vi "Update Armed.vi"(8 "error in (no error)":errorcluster, 10 "Armed":bool, 11 "Monitor-Pulse in":refnum<class "LabActor.lvclass">) -> (0 "error out":errorcluster, 3 "Monitor-Pulse out":refnum<class "LabActor.lvclass">)   [LabVIEW 2016, in "LabActor.lvclass"]
uses:
  LabActor.lvclass
  C:/github/LabActor/Controllers/Application Controller/Application Controller.lvclass
  Controllers/Application Controller/Application Controller.lvclass/Application Controller.ctl
  Controllers/Application Controller/Read Armed ref.vi
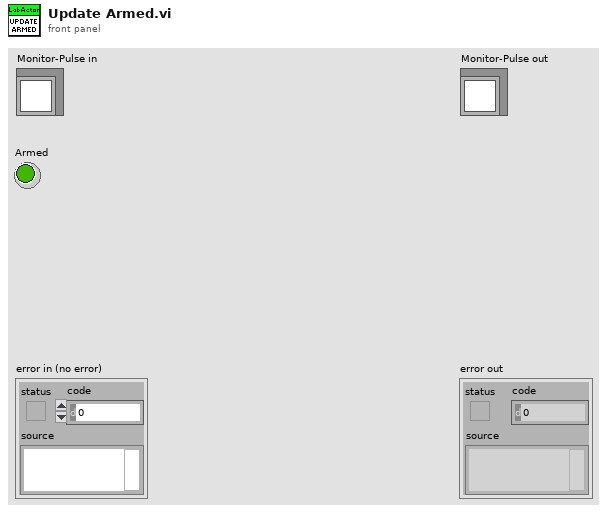
[diagram p1: front panel]
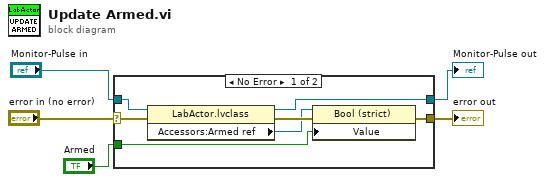
[diagram p0: block diagram]
diagram:
  n1 = case shown="No Error" "error in (no error)" {
    selector: "error in (no error)" -> [w11 w14]
    tunnel: [w10 w14] -> w4
    tunnel: [w7 w13] -> w2
    tunnel: "Monitor-Pulse in" -> [w8 w13]
    tunnel: "Armed" -> [w12 _]
    frame No Error {
      n2 = property class="LabActor.lvclass"(reference=w8, error in=w11) -> (reference out=w7:refnum<class "LabActor.lvclass">, error out=w9:errorcluster, "Accessors:Armed ref"=w6:refnum<vi>)
      n3 = property class="Bool (strict)"(reference=w6, error in=w9, "Value"=w12) -> (error out=w10:errorcluster)  [unwired: 1 out]
    }
    frame Error {
    }
  }
  "error out" <- w4
  "Monitor-Pulse out" <- w2
